vi "HWConfigSelected.vi"(8 "error in (no error)":errorcluster, 11 "StaticOutputEditor in":refnum<class "StaticOutputEditor.lvclass">) -> (0 "error out":errorcluster, 3 "StaticOutputEditor out":refnum<class "StaticOutputEditor.lvclass">)   [LabVIEW 2011, in "Views.lvlib" / "ScriptEditor.lvlib" / "StaticOutputEditor.lvclass"]
uses:
  StaticOutputEditor.lvclass
  StaticOutputEditor.lvclass/StaticOutputEditor.ctl
  Tools/DatabaseHelpers/Database Objects/HWConfiguration/HWConfigurations.lvclass
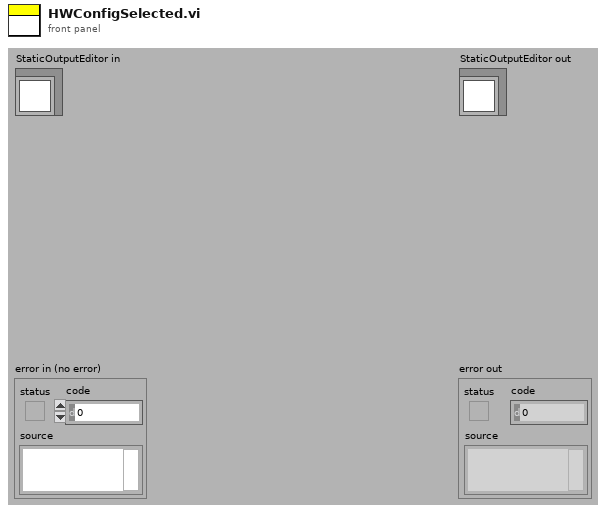
[diagram p1: front panel]
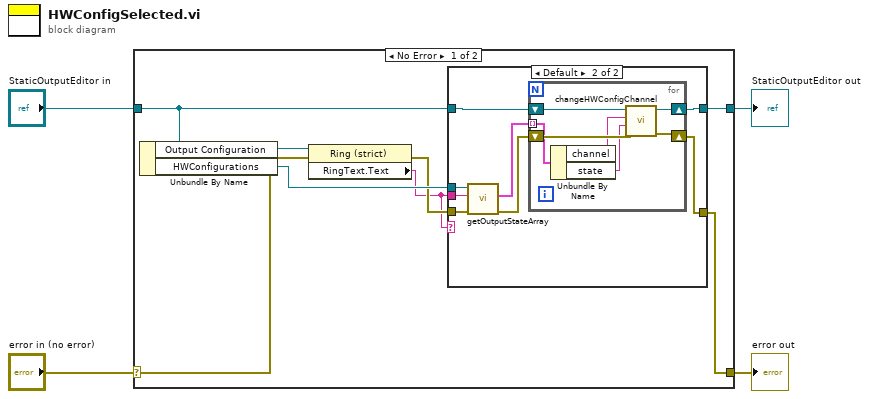
[diagram p0: block diagram]
diagram:
  n1 = case shown="No Error" "error in (no error)" {
    selector: "error in (no error)" -> [w9 w31]
    tunnel: [w5 w31] -> w3
    tunnel: [w6 w30] -> w1
    tunnel: "StaticOutputEditor in" -> [w7 w30]
    frame No Error {
      n2 = Unbundle By Name(w7) -> ("Output Configuration"=w12:refnum<vi>, "HWConfigurations"=w11:refnum<class "HWConfigurations.lvclass">)
      n3 = property class="Ring (strict)"(reference=w12, error in=w9) -> (error out=w10:errorcluster, "RingText.Text"=w8:string)  [unwired: 1 out]
      n4 = case shown="Default" w8 {
        tunnel: w8 -> [_ w22]
        tunnel: w11 -> [_ w21]
        tunnel: w10 -> [w13 w20]
        tunnel: w7 -> [w14 w19]
        tunnel: [w14 w18] -> w6
        tunnel: [w13 w15] -> w5
        frame "" {
        }
        frame Default {
          n5 = call "getOutputStateArray.vi"("error in (no error)"=w20, "configuration_name"=w22, "HWConfiguration in"=w21) -> ("error out"=w17:errorcluster, "outputStateArray"=w16:cluster{"channel":string, "state":string}[])  [unwired: 6 in, 1 out]
          n6 = for {
            tunnel: w16 -> [w26] mode=indexing
            shift-right: [w25] -> w15
            shift-left: w17 -> [w27]
            shift-right: [w28] -> w18
            shift-left: w19 -> [w29]
            n7 = Unbundle By Name(w26) -> ("channel"=w23:string, "state"=w24:string)
            n8 = call "changeHWConfigChannel.vi"("error in (no error)"=w27, "state"=w24, "channel"=w23, "StaticOutputEditor in"=w29) -> ("error out"=w25:errorcluster, "StaticOutputEditor out"=w28:refnum<class "StaticOutputEditor.lvclass">)  [unwired: 6 in]
          }
        }
      }
    }
    frame Error {
    }
  }
  "error out" <- w3
  "StaticOutputEditor out" <- w1
